vi "Build Tree Tag.vi"(8 "error in":errorcluster, 11 "LabVIEWItem in":refnum<class "LabVIEWItem.lvclass">) -> (0 "error out":errorcluster, 2 "Tree Tag":string)   [LabVIEW 2019, in "Panther Dashboard.lvlib" / "LabVIEWItem.lvclass"]
uses:
  LabVIEWItem.lvclass
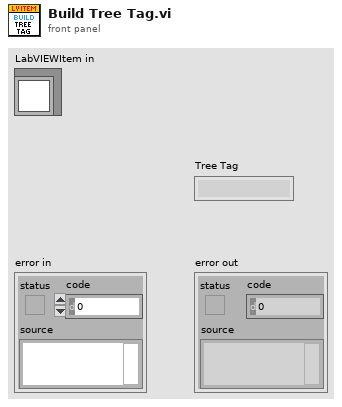
[diagram p1: front panel]
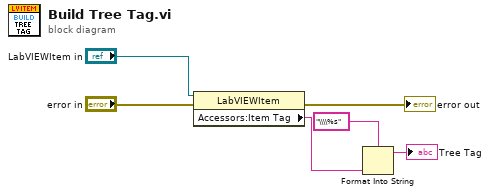
[diagram p0: block diagram]
diagram:
  n1 = property class="LabVIEWItem"(reference="LabVIEWItem in", error in="error in") -> (error out=→"error out":errorcluster, "Accessors:Item Tag"=w2:string)  [unwired: 1 out]
  n2 = Format Into String(format string="\\\\%s", w2) -> (resulting string=→"Tree Tag":string)  [unwired: 2 in, 1 out]
